vi "State Machine.vi"(8 "error in (no error)":errorcluster) -> (0 "error out":errorcluster)   [LabVIEW 2018]
uses:
  State Machine/State Machine.lvclass
  State Machine/State Machine.lvclass/State Machine.ctl
  <vilib>/addons/_JKI Toolkits/Caraya/classes/Test/Test.lvclass
  <vilib>/addons/_JKI Toolkits/Caraya/classes/Assert/Assert.lvclass
panel:
  in  "State Machine in 2":refnum<class "State Machine.lvclass">
  in  "State Machine in":refnum<class "State Machine.lvclass">
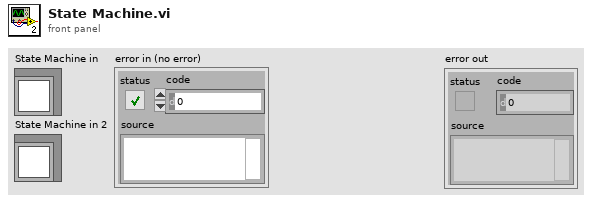
[diagram p1: front panel]
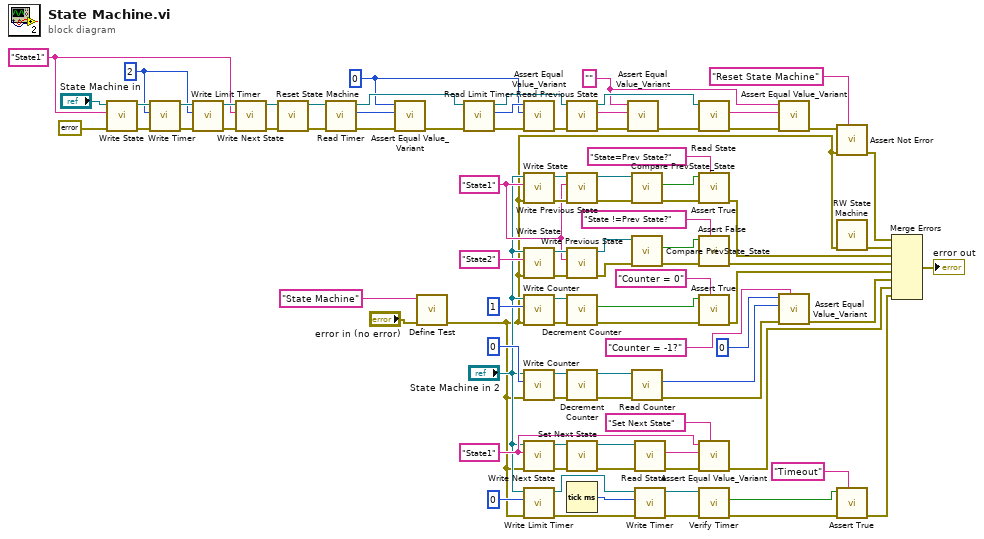
[diagram p0: block diagram]
diagram:
  w15 = "State1" ("Label (VI Title)")
  w24 = "" ("State")
  w31 = u16 0 ("Counter")
  w47 = u16 2 ("Counter")
  w48 = "State1" ("Label (VI Title)")
  w73 = "State1" ("Label (VI Title)")
  n1 = call-dynamic "Write State.vi"("error in (no error)"=errorcluster {"status"=FALSE, "code"=0, "source"=""}, "State"=w48, "State Machine in"="State Machine in") -> ("error out"=w52:errorcluster, "State Machine out"=w51:refnum<class "State Machine.lvclass">)  [unwired: 7 in]
  n2 = call "Write Timer.vi"("error in (no error)"=w52, "Timer"=w47, "State Machine in"=w51) -> ("error out"=w53:errorcluster, "State Machine out"=w50:refnum<class "State Machine.lvclass">)  [unwired: 7 in]
  n3 = call "Write Limit Timer.vi"("error in (no error)"=w53, "Limit Timer"=w47, "State Machine in"=w50) -> ("error out"=w54:errorcluster, "State Machine out"=w49:refnum<class "State Machine.lvclass">)  [unwired: 7 in]
  n4 = call "Write Next State.vi"("error in (no error)"=w54, "Next State"=w48, "State Machine in"=w49) -> ("error out"=w46:errorcluster, "State Machine out"=w45:refnum<class "State Machine.lvclass">)  [unwired: 7 in]
  n5 = call "Reset State Machine.vi"("error in (no error)"=w46, "State Machine in"=w45) -> ("error out"=w40:errorcluster, "State Machine out"=w41:refnum<class "State Machine.lvclass">)  [unwired: 8 in]
  n6 = call "Read Timer.vi"("error in (no error)"=w40, "State Machine in"=w41) -> ("error out"=w39:errorcluster, "Timer"=w37:u32, "State Machine out"=w42:refnum<class "State Machine.lvclass">)  [unwired: 7 in]
  n7 = call <vilib>:"Assert Equal Value_Variant.vi"("error in (no error)"=w39, "Y"=w37, "X"=w31) -> ("error out"=w38:errorcluster)  [unwired: 7 in, 1 out]
  n8 = call <vilib>:"Define Test.vi"("error in (no error)"="error in (no error)", "Label (VI Title)"="State Machine") -> ("error out"=w10:errorcluster)  [unwired: 8 in, 1 out]
  n9 = call "Read Limit Timer.vi"("error in (no error)"=w38, "State Machine in"=w42) -> ("error out"=w33:errorcluster, "Limit Timer"=w32:u32, "State Machine out"=w43:refnum<class "State Machine.lvclass">)  [unwired: 7 in]
  n10 = call <vilib>:"Assert Equal Value_Variant.vi"("error in (no error)"=w33, "Y"=w31, "X"=w32) -> ("error out"=w34:errorcluster)  [unwired: 7 in, 1 out]
  n11 = call-dynamic "Write State.vi"("error in (no error)"=w10, "State"=w73, "State Machine in"="State Machine in 2") -> ("error out"=w90:errorcluster, "State Machine out"=w89:refnum<class "State Machine.lvclass">)  [unwired: 7 in]
  n12 = call-dynamic "Write State.vi"("error in (no error)"=w10, "State"="State2" ("Label (VI Title)"), "State Machine in"="State Machine in 2") -> ("error out"=w75:errorcluster, "State Machine out"=w76:refnum<class "State Machine.lvclass">)  [unwired: 7 in]
  n13 = call "Write Counter.vi"("error in (no error)"=w10, "Counter"=u16 1, "State Machine in"="State Machine in 2") -> ("error out"=w70:errorcluster, "State Machine out"=w69:refnum<class "State Machine.lvclass">)  [unwired: 7 in]
  n14 = call "Write Counter.vi"("error in (no error)"=w10, "Counter"=u16 0, "State Machine in"="State Machine in 2") -> ("error out"=w63:errorcluster, "State Machine out"=w64:refnum<class "State Machine.lvclass">)  [unwired: 7 in]
  n15 = call "Write Next State.vi"("error in (no error)"=w10, "Next State"=w15, "State Machine in"="State Machine in 2") -> ("error out"=w22:errorcluster, "State Machine out"=w21:refnum<class "State Machine.lvclass">)  [unwired: 7 in]
  n16 = call "Write Limit Timer.vi"("error in (no error)"=w10, "Limit Timer"=u32 0, "State Machine in"="State Machine in 2") -> ("error out"=w3:errorcluster, "State Machine out"=w2:refnum<class "State Machine.lvclass">)  [unwired: 7 in]
  n17 = call-dynamic "Read Previous State.vi"("error in (no error)"=w34, "State Machine in"=w43) -> ("error out"=w30:errorcluster, "Previous State"=w25:string, "State Machine out"=w44:refnum<class "State Machine.lvclass">)  [unwired: 7 in]
  n18 = call-dynamic "Write Previous State.vi"("error in (no error)"=w90, "Previous State"=w73, "State Machine in"=w89) -> ("error out"=w91:errorcluster, "State Machine out"=w88:refnum<class "State Machine.lvclass">)  [unwired: 7 in]
  n19 = call-dynamic "Write Previous State.vi"("error in (no error)"=w75, "Previous State"=w73, "State Machine in"=w76) -> ("error out"=w74:errorcluster, "State Machine out"=w77:refnum<class "State Machine.lvclass">)  [unwired: 7 in]
  n20 = call "Decrement Counter.vi"("error in (no error)"=w70, "State Machine in"=w69) -> ("error out"=w68:errorcluster, "counter = zero"=w65:bool)  [unwired: 7 in, 1 out]
  n21 = call "Decrement Counter.vi"("error in (no error)"=w63, "State Machine in"=w64) -> ("error out"=w61:errorcluster, "State Machine out"=w60:refnum<class "State Machine.lvclass">)  [unwired: 7 in, 1 out]
  n22 = call "Set Next State.vi"("error in (no error)"=w22, "State Machine in"=w21) -> ("error out"=w19:errorcluster, "State Machine out"=w18:refnum<class "State Machine.lvclass">)  [unwired: 8 in]
  n23 = Tick Count (ms)() -> (millisecond timer value=w1:u32)
  n24 = call <vilib>:"Assert Equal Value_Variant.vi"("error in (no error)"=w30, "Y"=w25, "X"=w24) -> ("error out"=w29:errorcluster)  [unwired: 7 in, 1 out]
  n25 = call "Compare PrevState_State.vi"("error in (no error)"=w91, "State Machine in"=w88) -> ("error out"=w85:errorcluster, "prev = state ?"=w83:bool)  [unwired: 7 in, 1 out]
  n26 = call "Compare PrevState_State.vi"("error in (no error)"=w74, "State Machine in"=w77) -> ("error out"=w78:errorcluster, "prev = state ?"=w80:bool)  [unwired: 7 in, 1 out]
  n27 = call "Read Counter.vi"("error in (no error)"=w61, "State Machine in"=w60) -> ("error out"=w57:errorcluster, "Counter"=w59:u16)  [unwired: 7 in, 1 out]
  n28 = call-dynamic "Read State.vi"("error in (no error)"=w19, "State Machine in"=w18) -> ("error out"=w17:errorcluster, "State"=w16:string)  [unwired: 7 in, 1 out]
  n29 = call "Write Timer.vi"("error in (no error)"=w3, "Timer"=w1, "State Machine in"=w2) -> ("error out"=w5:errorcluster, "State Machine out"=w4:refnum<class "State Machine.lvclass">)  [unwired: 7 in]
  n30 = call-dynamic "Read State.vi"("error in (no error)"=w29, "State Machine in"=w44) -> ("error out"=w28:errorcluster, "State"=w26:string)  [unwired: 7 in, 1 out]
  n31 = call <vilib>:"Assert True.vi"("Label"="State=Prev State?", "error in (no error)"=w85, "True?"=w83) -> ("error out"=w84:errorcluster)  [unwired: 7 in, 1 out]
  n32 = call <vilib>:"Assert False.vi"("Label"="State !=Prev State?", "error in (no error)"=w78, "False?"=w80) -> ("error out"=w72:errorcluster)  [unwired: 7 in, 1 out]
  n33 = call <vilib>:"Assert True.vi"("Label"="Counter = 0", "error in (no error)"=w68, "True?"=w65) -> ("error out"=w66:errorcluster)  [unwired: 7 in, 1 out]
  n34 = call <vilib>:"Assert Equal Value_Variant.vi"("Label"="Set Next State", "error in (no error)"=w17, "Y"=w16, "X"=w15) -> ("error out"=w13:errorcluster)  [unwired: 6 in, 1 out]
  n35 = call "Verify Timer.vi"("error in (no error)"=w5, "State Machine in"=w4) -> ("error out"=w9:errorcluster, "time out"=w6:bool)  [unwired: 7 in, 1 out]
  n36 = call <vilib>:"Assert Equal Value_Variant.vi"("error in (no error)"=w28, "Y"=w26, "X"=w24) -> ("error out"=w27:errorcluster)  [unwired: 7 in, 1 out]
  n37 = call <vilib>:"Assert Equal Value_Variant.vi"("Label"="Counter = -1?", "error in (no error)"=w57, "Y"=w59, "X"=u16 0 ("Counter")) -> ("error out"=w56:errorcluster)  [unwired: 6 in, 1 out]
  n38 = call <vilib>:"Assert Not Error.vi"("Label"="Reset State Machine", "error in (no error)"=w10, "Not Error?"=w27) -> ("error out"=w36:errorcluster)  [unwired: 7 in, 1 out]
  n39 = call "RW State Machine.vi"("error in (no error)"=w10) -> ("error out"=w87:errorcluster)  [unwired: 10 in]
  n40 = call <vilib>:"Assert True.vi"("Label"="Timeout", "error in (no error)"=w9, "True?"=w6) -> ("error out"=w8:errorcluster)  [unwired: 7 in, 1 out]
  n41 = Merge Errors(w36, w87, w84, w72, w66, w56, w13, w8) -> (→"error out":errorcluster)
